vi "Invert Selection.vi"(0 "Display State In":T2, 9 "Container State":T1, 11 "error in (no error)":errorcluster) -> (4 "Display State Out":T2, 15 "error out":errorcluster)   [LabVIEW 2014, in "ListBox XControl.xctl"]
uses:
  ListBox XControl.xctl
  <vilib>/_xctls/Container State.ctl
  State ListBox.ctl
  <vilib>/_xctls/XControlSupport.lvlib
panel:
  in  "Container State 2":T1
  # "Add Controls & Indicators that form the parameters of the method here. Hook them to the connector pane. Do not delete the controls & indicators that are already hooked to the connector pane.\n \nTo setup the parameters  for this method, right click on this item in the Project Tree & select \"Configure Method...\"."
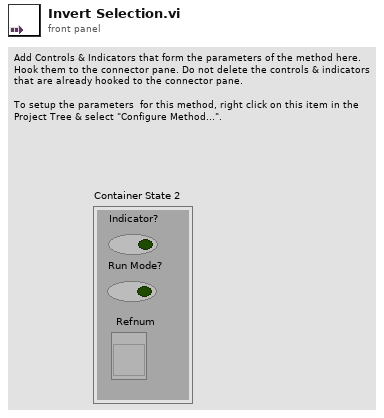
[diagram p1: front panel]
types:
  T1 = typedef "XControlSupport.lvlib/Container State.ctl" = cluster{"Indicator?":bool, "Run Mode?":bool, " Refnum":refnum<vi>}
  T2 = typedef "ListBox XControl.xctl/State ListBox.ctl" = cluster{"ItemNames[]":string[], "Listbox Ref":refnum<vi>, "Select All By Default":bool}
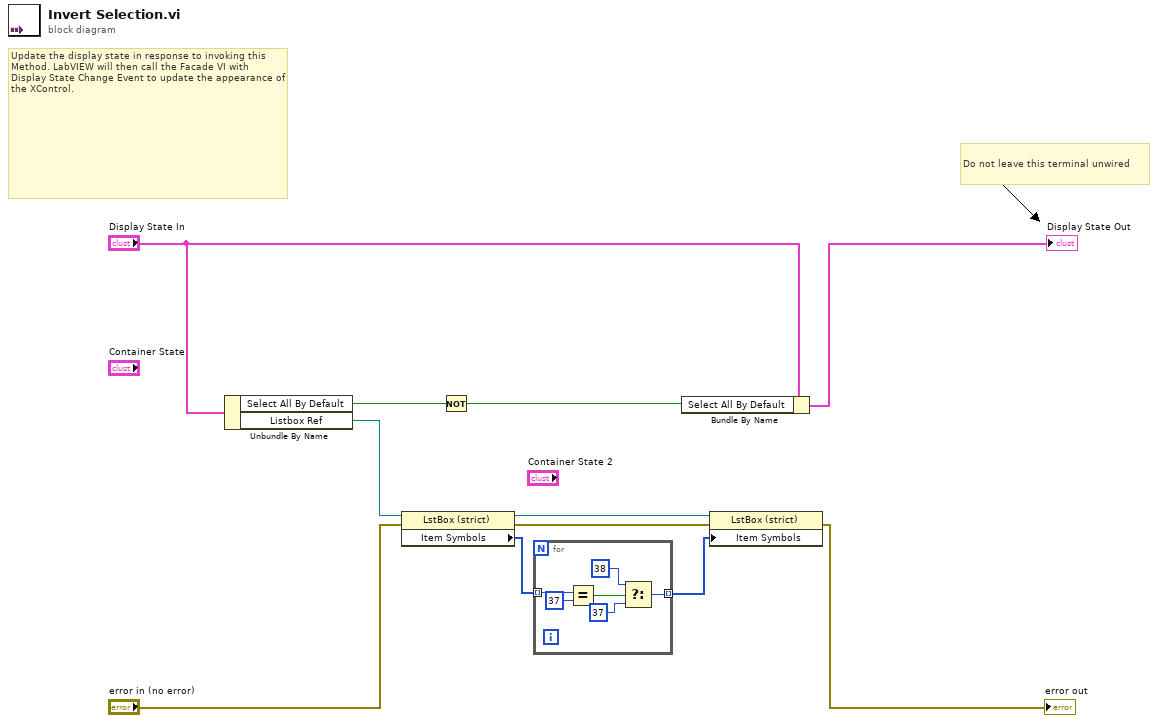
[diagram p0: block diagram]
diagram:
  # "Do not leave this terminal unwired"
  # "Update the display state in response to invoking this Method. LabVIEW will then call the Facade VI with Display State Change Event to update the appearance of the XControl."
  n1 = Unbundle By Name("Display State In") -> ("Select All By Default"=w11:bool, "Listbox Ref"=w6:refnum<vi>)
  n2 = property class="LstBox (strict)"(reference=w6, error in="error in (no error)") -> (reference out=w5:refnum<vi>, error out=w7:errorcluster, "Item Symbols"=w1:i32[])
  n3 = Not(x=w11) -> (.not. x?=w10:bool)
  n4 = for {
    tunnel: [w15] -> w2 mode=indexing
    tunnel: w1 -> [w14] mode=indexing
    n5 = Equal?(x=w14, y=37) -> (x = y?=w12:bool)
    n6 = Select(t=38, s=w12, f=37) -> (s? t:f=w15:i32)
  }
  n7 = Bundle By Name(cluster="Display State In", "Select All By Default"=w10) -> (→"Display State Out":T2)
  n8 = property class="LstBox (strict)"(reference=w5, error in=w7, "Item Symbols"=w2) -> (error out=→"error out":errorcluster)  [unwired: 1 out]
